vi "Get_APC_Limit_for_Sweep.vi"(8 "error in (no error)":errorcluster, 9 "maxwave":dbl, 10 "minwave":dbl, 11 ".NET Reference in":refnum<k24>) -> (0 "error out":errorcluster, 1 "maxpower":sgl, 3 "Reference out":refnum<k24>)   [LabVIEW 2017]
uses:
  LV_IL_Sample/DLL/InstrumentDLL.dll
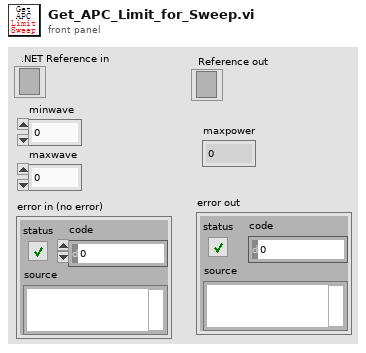
[diagram p1: front panel]
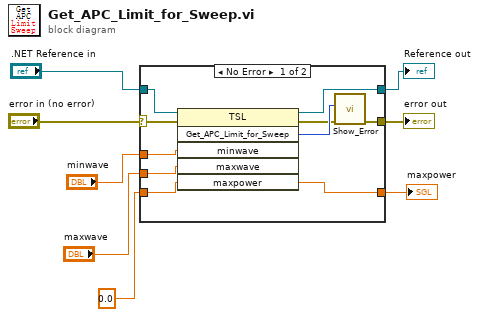
[diagram p0: block diagram]
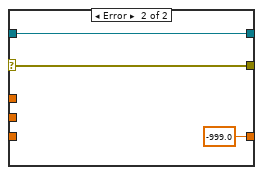
[diagram p2: hidden frame]
diagram:
  n1 = case shown="No Error" "error in (no error)" {
    selector: "error in (no error)" -> [w13 w21]
    tunnel: ".NET Reference in" -> [w18 w20]
    tunnel: [w17 w20] -> w7
    tunnel: [w14 w21] -> w6
    tunnel: "minwave" -> [w12 _]
    tunnel: "maxwave" -> [w11 _]
    tunnel: sgl 0.0 ("maxpower") -> [w10 _]
    tunnel: [w9 -999.0 ("maxpow")] -> w1
    frame No Error {
      n2 = invoke on="调用节点" class="TSL" method="Get_APC_Limit_for_Sweep"(reference=w18, error in=w13, "minwave"=w12, "maxwave"=w11, "maxpower"=w10) -> (reference out=w17:refnum<k24>, error out=w15:errorcluster, "Get_APC_Limit_for_Sweep"=w16:i32, "maxpower"=w9:sgl)  [unwired: 1 in, 2 out]
      n3 = call "Show_Error.vi"("error in (no error)"=w15, "Error"=w16) -> ("error out"=w14:errorcluster)  [unwired: 9 in]
    }
    frame Error {
    }
  }
  "Reference out" <- w7
  "error out" <- w6
  "maxpower" <- w1
